vi "EKSPERIMENT.vi"() -> ()   [LabVIEW 2013]
panel:
  out "NAPON":dynamicdata(graph)
  out "Izlazni napon u V":dbl
  out "Izmjerena udaljenost u cm":dbl
  in  "Stop":bool
  in  "Start":bool
  in  "Trajanje akvizicije u sec.":dbl
  in  "Broj semplova u sec.":dbl
  out "DUŽINA":dynamicdata(graph)
  out "TRAJANJE IMPULSA":dynamicdata(graph)
  out "Vrijeme pulsa u us":dbl
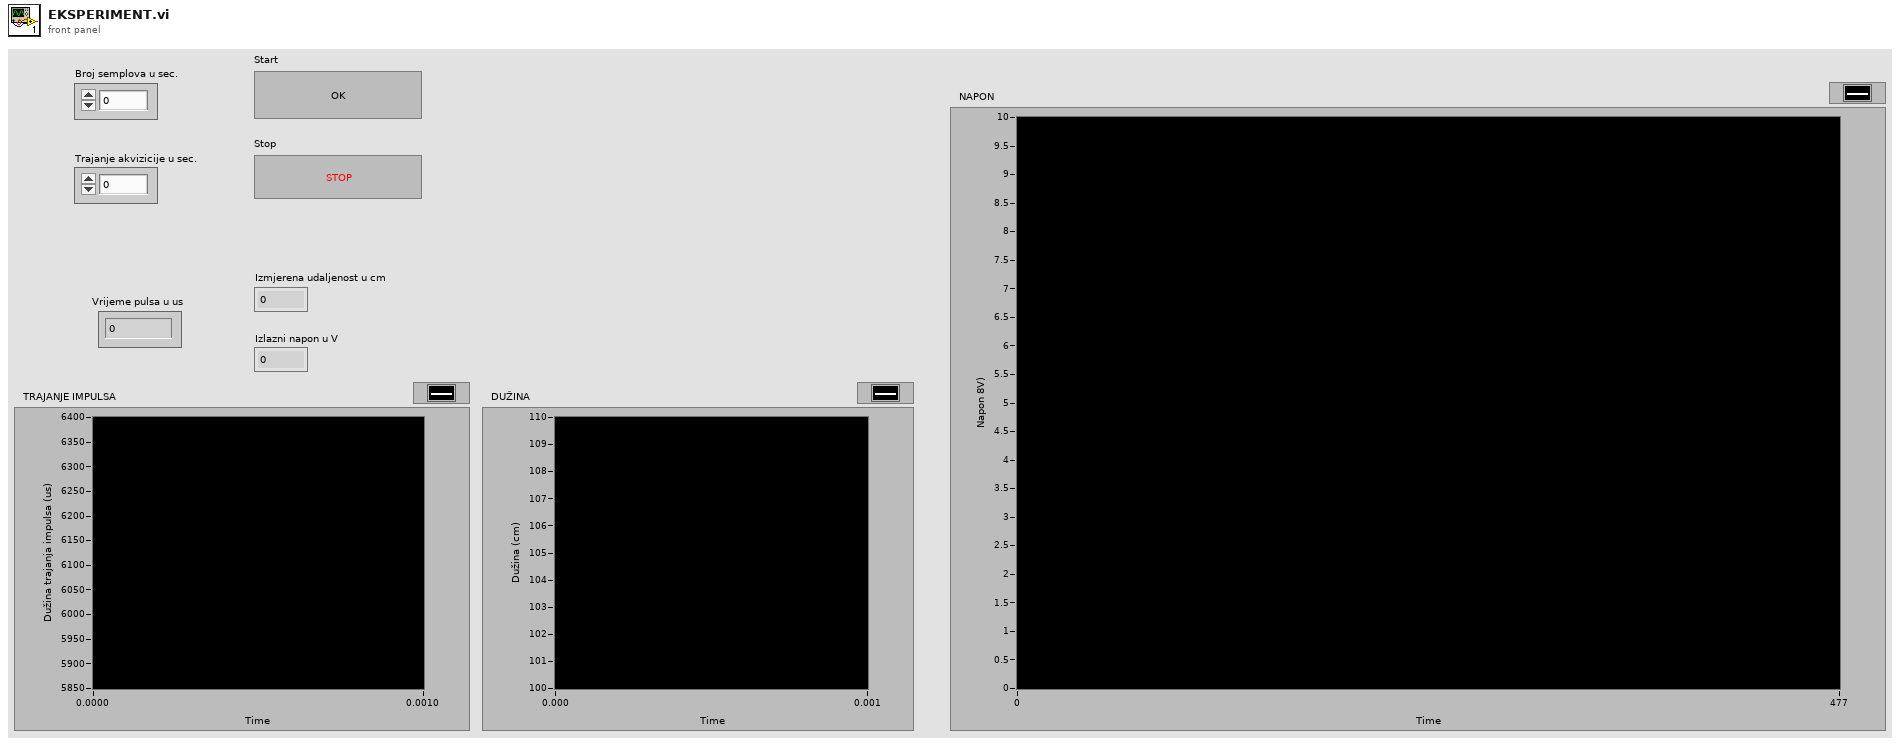
[diagram p1: front panel]
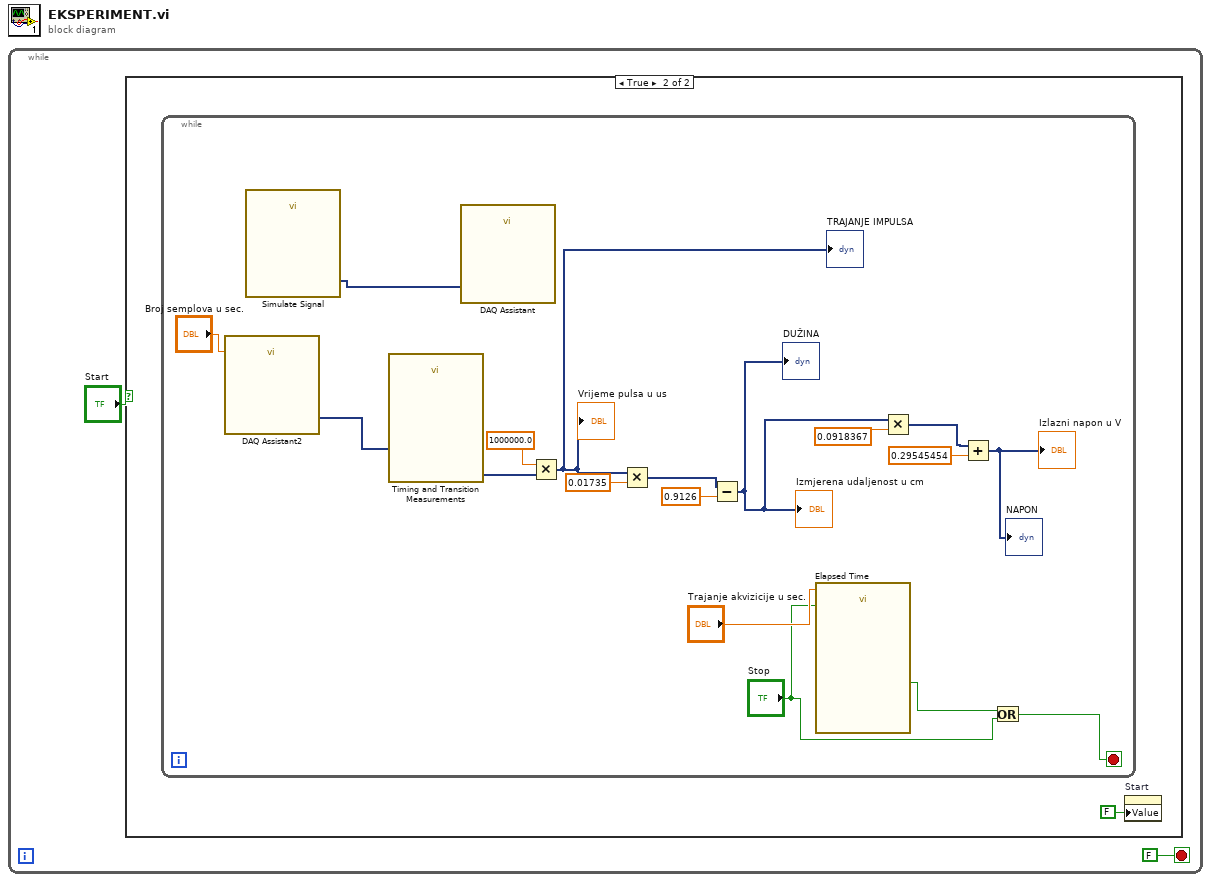
[diagram p0: block diagram]
diagram:
  n1 = while {
    stop <- FALSE stop-if-true
    n2 = case shown="True" "Start" {
      frame False {
      }
      frame True {
        n3 = while {
          stop <- w13 stop-if-true
          n4 = call "DAQ Assistant2"("number of samples"="Broj semplova u sec.") -> ("data"=w18:dynamicdata)  [unwired: 16 in, 2 out]
          n5 = call "Simulate Signal"() -> ("Square"=w19:dynamicdata)  [unwired: 14 in, 1 out]
          n6 = call "Timing and Transition Measurements"("Signals"=w18) -> ("Duration"=w21:dynamicdata)  [unwired: 9 in, 1 out]
          n7 = call "DAQ Assistant"("data"=w19) -> ()  [unwired: 17 in, 2 out]
          n8 = Multiply(x=1000000.0, y=w21) -> (x*y=w9:dynamicdata)
          "Vrijeme pulsa u us" <- w9
          "TRAJANJE IMPULSA" <- w9
          n9 = Multiply(x=w9, y=0.01735) -> (x*y=w11:dynamicdata)
          n10 = Subtract(x=w11, y=0.9126) -> (x-y=w8:dynamicdata)
          "DUŽINA" <- w8
          "Izmjerena udaljenost u cm" <- w8
          n11 = call "Elapsed Time"("Time Target (s)"="Trajanje akvizicije u sec.", "Reset"="Stop") -> ("Time has Elapsed"=w15:bool)  [unwired: 10 in, 7 out]
          n12 = Multiply(x=w8, y=0.0918367) -> (x*y=w6:dynamicdata)
          n13 = Add(x=w6, y=0.29545454) -> (x+y=→"Izlazni napon u V" →"NAPON":dynamicdata)
          n14 = Or(x=w15, y="Stop") -> (x .or. y?=w13:bool)
        }
        n15 = property on="Start" class="Bool (strict)"("Value"=FALSE ("Start")) -> ()  [unwired: 2 in, 2 out]
      }
    }
  }
